vi "Create Folder Index.vi"(8 "error in (no error)":errorcluster, 10 "File or Folder Path":path, 11 "All Files in Dir":path[](array[path])) -> (0 "error out":errorcluster)   [LabVIEW 2016, in "LV to ITX.lvclass"]
uses:
  LV to ITX.lvclass
  <vilib>/Utility/file.llb/Write Delimited Spreadsheet (string).vi
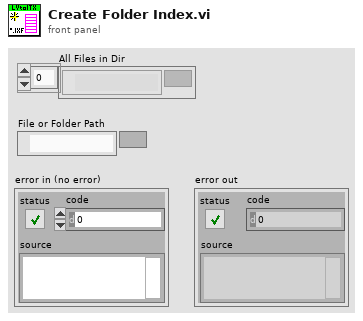
[diagram p1: front panel]
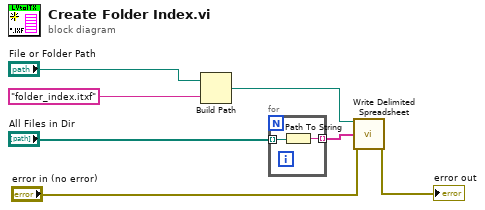
[diagram p0: block diagram]
diagram:
  n1 = Build Path(base path="File or Folder Path", name or relative path="folder_index.itxf") -> (appended path=w4:path)
  n2 = for {
    tunnel: "All Files in Dir" -> [w8] mode=indexing
    tunnel: [w9] -> w3 mode=indexing
    n3 = Path To String(path=w8) -> (string=w9:string)
  }
  n4 = call-poly <vilib>:"Write Delimited Spreadsheet.vi"("file path (dialog if empty)"=w4, "1D data"=w3, "error in (no error)"="error in (no error)") -> ("error out"=→"error out":errorcluster)  [unwired: 11 in, 1 out]
